vi "单步控制界面.vi"(11 "当前瓶号":u16) -> ()   [LabVIEW 2016, in "超标留样集成.lvlib" / "ESTD1200.lvlib"]
uses:
  ESTD1200.lvlib
panel:
  in  "关闭":bool
  in  "排空当前瓶":bool
  in  "选择留样瓶":bool
  in  "排空留样瓶":bool
  # "单步调试"
  # "只在待机时启动有效"
  # "只在待机时启动有效"
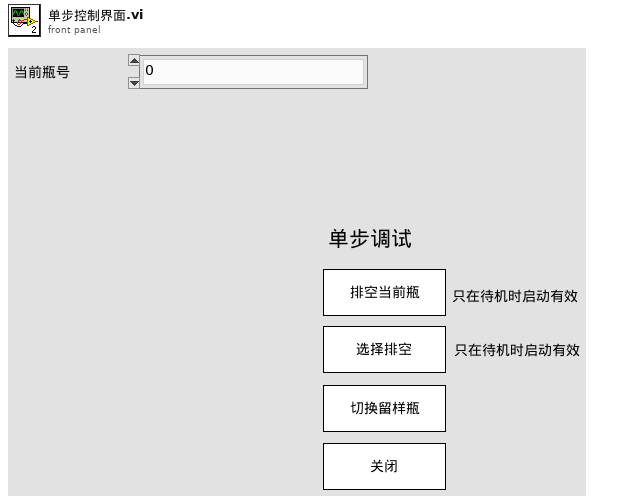
[diagram p1: front panel]
types:
  T1 = enum16{"open", "read", "write", "write single", "close"}
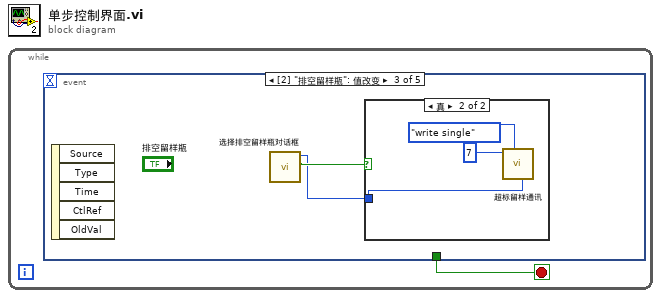
[diagram p0: block diagram]
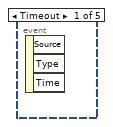
[diagram p2: hidden frame]
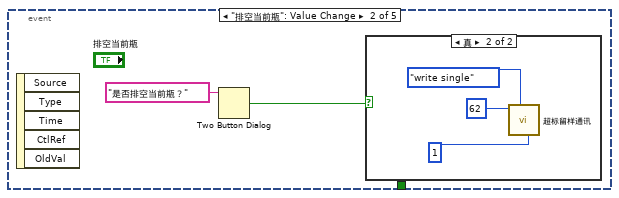
[diagram p3: hidden frame]
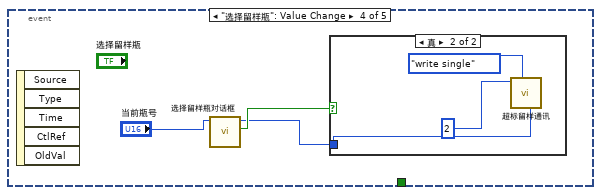
[diagram p6: hidden frame]
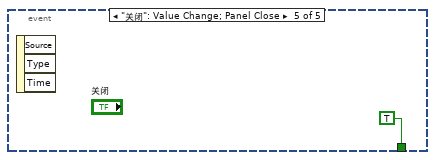
[diagram p8: hidden frame]
diagram:
  n1 = while {
    stop <- w1 stop-if-true
    n2 = event shown="[2] \"排空留样瓶\": 值改变" {
      selector: _ -> [_ _ _ _ _]
      dyn-events: _ -> [_ _ _ _ _]
      timeout: _ -> [_ _ _ _ _]
      tunnel: [_ _ _ _ TRUE] -> w1
      event Timeout {
        n3 = event-data() -> ()  [unwired: 1 in, 3 out]
      }
      event "排空当前瓶": Value Change {
        n4 = event-data() -> ()  [unwired: 1 in, 5 out]
        n5 = Two Button Dialog(message="是否排空当前瓶？" ("消息")) -> (T button?=w2:bool)  [unwired: 2 in]
        n6 = case shown="真" w2 {
          frame False {
          }
          frame True {
            n7 = call "超标留样通讯.vi"(4:u16 1 ("新元素/子数组"), 7:T1."write single" ("STEP"), 11:62 ("索引")) -> ()  [unwired: 7 in, 2 out]
          }
        }
      }
      event "排空留样瓶": Value Change {
        n8 = event-data() -> ()  [unwired: 1 in, 5 out]
        n9 = call "选择排空留样瓶对话框.vi"() -> ("布尔"=w8:bool, "选择留样瓶 2"=w7:u16)  [unwired: 10 in]
        n10 = case shown="真" w8 {
          tunnel: w7 -> [_ w9]
          frame False {
          }
          frame True {
            n11 = call "超标留样通讯.vi"(4:w9, 7:T1."write single" ("STEP"), 11:7 ("索引")) -> ()  [unwired: 7 in, 2 out]
          }
        }
      }
      event "选择留样瓶": Value Change {
        n12 = event-data() -> ()  [unwired: 1 in, 5 out]
        n13 = call "选择留样瓶对话框.vi"("选择留样瓶"="当前瓶号") -> ("布尔"=w14:bool, "选择留样瓶 2"=w13:u16)  [unwired: 9 in]
        n14 = case shown="真" w14 {
          tunnel: w13 -> [_ w15]
          frame False {
          }
          frame True {
            n15 = call "超标留样通讯.vi"(4:w15, 7:T1."write single" ("STEP"), 11:2 ("索引")) -> ()  [unwired: 7 in, 2 out]
          }
        }
      }
      event "关闭": Value Change; Panel Close {
        n16 = event-data() -> ()  [unwired: 1 in, 3 out]
      }
    }
  }
